vi "change post build step.vi"(8 "error in (no error)":errorcluster, 10 "User Project":refnum<vi>, 11 "NIVS_CDW_MetaDataObj in":refnum<class "NIVS_ScriptedModuleTemplate_MetaDataObj.lvclass">) -> (0 "error out":errorcluster)   [LabVIEW 2014, in "NIVS_ScriptedModuleTemplate_MetaDataObj.lvclass"]
uses:
  NIVS_ScriptedModuleTemplate_MetaDataObj.lvclass
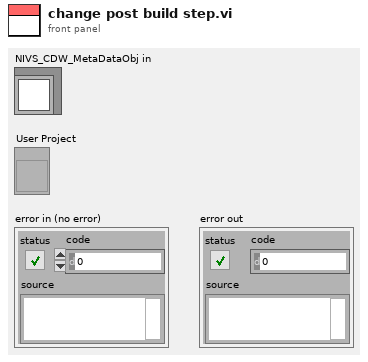
[diagram p1: front panel]
types:
  T1 = typedef "CD Wizard - Internal data.ctl" = cluster{"Common Information":cluster{"CD Name":string, "CD Target Folder":path, "CD Execution Mode":T2, "CD GUID":string}, "Extra Pages":T3[], "References":cluster{"System Explorer Library":refnum<vi>, "Shared Library":refnum<vi>, "Engine Library":refnum<vi>}, "Menu Settings":cluster{"Insert CD in submenu":bool, "Parent Menu Name":string}}
  T2 = typedef "CD Wizard - Execution Mode.ctl" = enum16{"Asynchronous", "Inline HW Interface", "Inline Model Interface", "Inline Timing and Sync", "Asynchronous Timing and Sync"}
  T3 = typedef "CD Wizard - Extra Page Name and GUID.ctl" = cluster{"Page Name":string, "Page GUID":string}
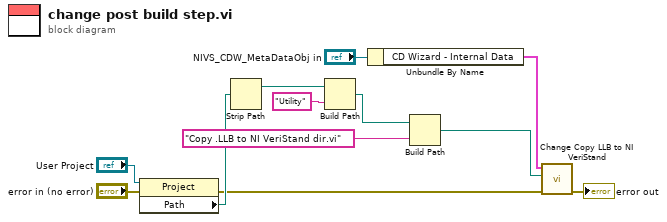
[diagram p0: block diagram]
diagram:
  n1 = property class="Project"(reference="User Project", error in="error in (no error)") -> (error out=w5:errorcluster, "Path"=w7:path)  [unwired: 1 out]
  n2 = Strip Path(path=w7) -> (stripped path=w9:path)  [unwired: 1 out]
  n3 = Build Path(base path=w9, name or relative path="Utility") -> (appended path=w8:path)
  n4 = Unbundle By Name("NIVS_CDW_MetaDataObj in") -> ("CD Wizard - Internal Data"=w2:T1)
  n5 = Build Path(base path=w8, name or relative path="Copy .LLB to NI VeriStand dir.vi") -> (appended path=w12:path)
  n6 = call "Change Copy LLB to NI VeriStand.vi"("error in (no error)"=w5, "Copy .LLB to ... path"=w12, "CD Wizard - Internal Data"=w2) -> ("error out"=→"error out":errorcluster)  [unwired: 8 in]
